vi "I2C and GPIO Timestamp Loop.vi"(0 "fpga interface in":refnum<k20>, 1 "'stop' notifier":refnum<notifier>, 2 "log to disk":bool=TRUE, 5 "tdms file directory":path, 7 "gpio to display":T2[](array[typedef])=[{"GPIO Bank"=enum."Ser0 GPIO Bank", "GPIO Number"=0}], 9 "timestamp filter":T1[](array[typedef])=[enum."User24", enum."User25", enum."User26", enum."User27", enum."User28", enum."User29", enum."User30", enum."User31"], 11 "error in (no error)":errorcluster) -> (4 "i2c data":string[][](array[string]), 6 "gpio timestamps waveform":digitalwaveform[](graph), 8 "error parsing gpio timestamps":bool, 15 "error out":errorcluster)   [LabVIEW 2023, in "GettingStarted_Common_148X_Host.lvlib"]
uses:
  GettingStarted_Common_148X_Host.lvlib
  <instrlib>/FlexRIO/CSI-2/v2/FPGA/Types/Timestamp ID.ctl
  <instrlib>/FlexRIO/CSI-2/v2/FPGA/NI CSI-2 API FPGA v2.lvlib
  Types/GPIO Filter.ctl
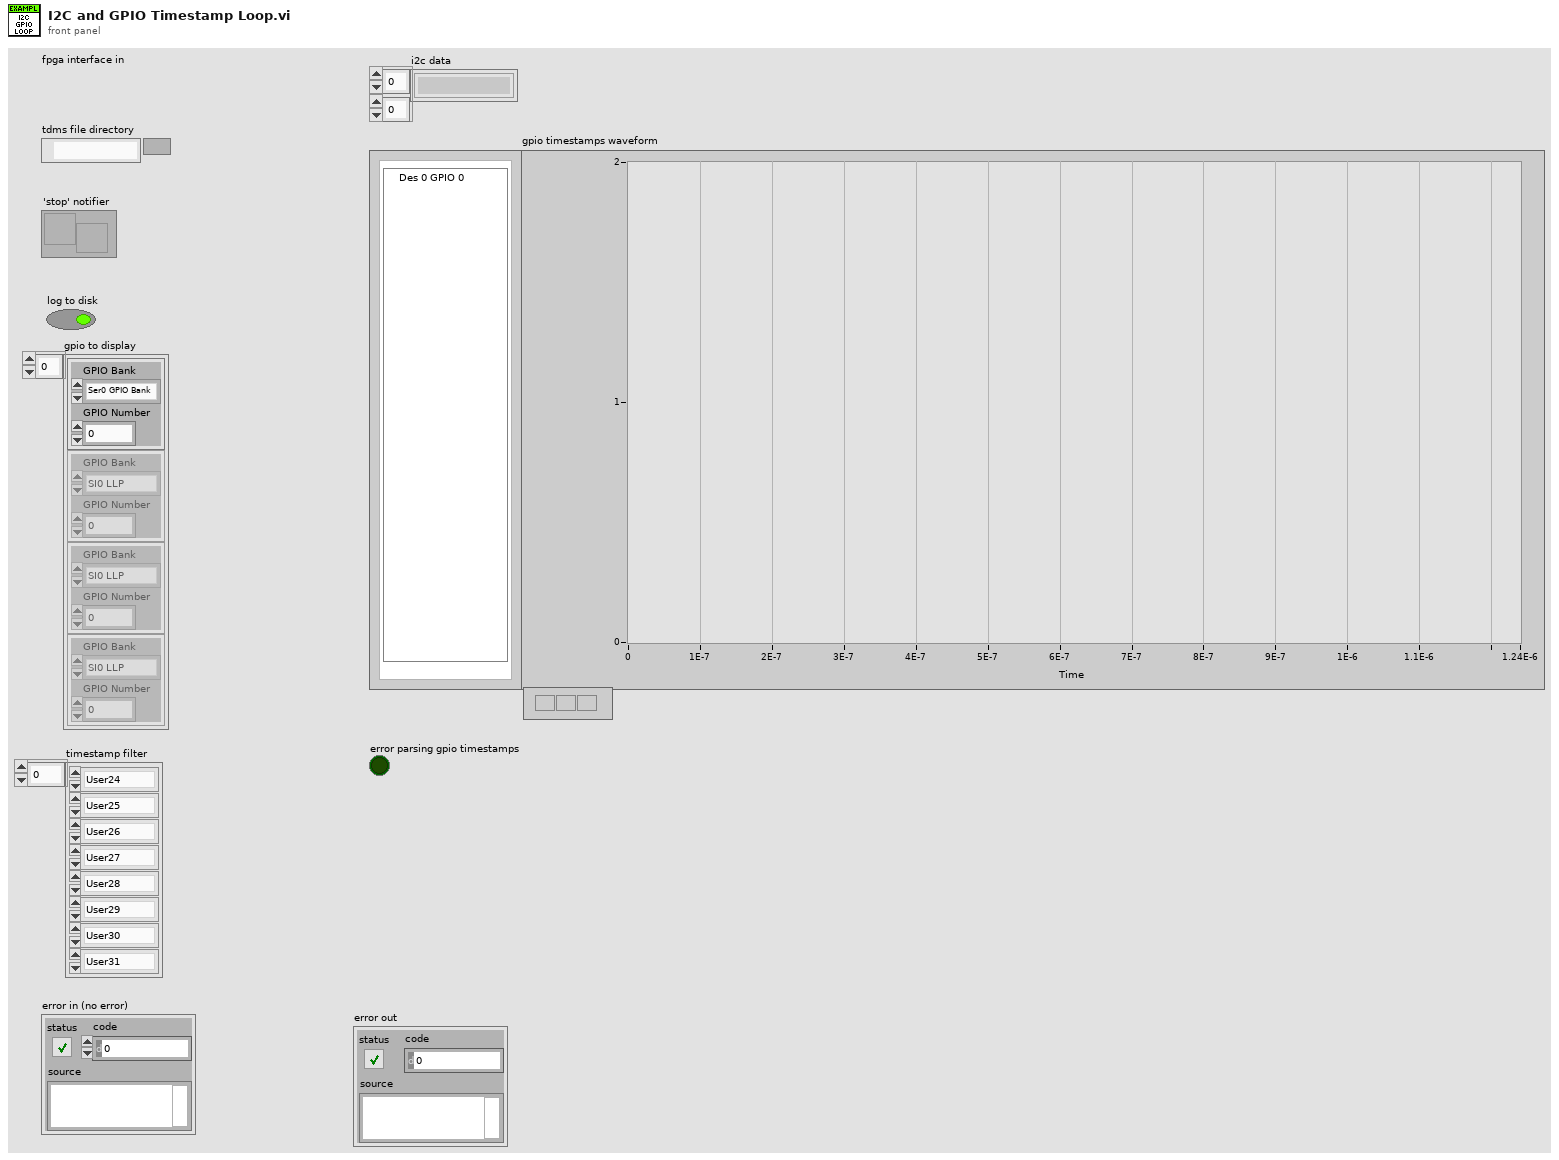
[diagram p1: front panel]
types:
  T1 = typedef "NI CSI-2 API FPGA v2.lvlib/Timestamp ID.ctl" = enum8{"SI0 LLP", "SI1 LLP", "SI2 LLP", "SI3 LLP", "SI4 LLP", "SI5 LLP", "SI6 LLP", "SI7 LLP", "SO0 LLP", "SO1 LLP", "SO2 LLP", "SO3 LLP", "SO4 LLP", "SO5 LLP", "SO6 LLP", "SO7 LLP", "Ser0 GPIO Bank", "Ser1 GPIO Bank", "Ser2 GPIO Bank", "Ser3 GPIO Bank", "Ser4 GPIO Bank", "Ser5 GPIO Bank", "Ser6 GPIO Bank", "Ser7 GPIO Bank", "Des0 GPIO Bank", "Des1 GPIO Bank", "Des2 GPIO Bank", "Des3 GPIO Bank", "Des4 GPIO Bank", "Des5 GPIO Bank", "Des6 GPIO Bank", "Des7 GPIO Bank", "User0", "User1", "User2", "User3", "User4", "User5", "User6", "User7", "User8", "User9", "User10", "User11", "User12", "User13", "User14", "User15", "User16", "User17", "User18", "User19", "User20", "User21", "User22", "User23", "User24", "User25", "User26", "User27", "User28", "User29", "User30", "User31"}
  T2 = typedef "GettingStarted_Common_148X_Host.lvlib/GPIO Filter.ctl" = cluster{"GPIO Bank":T1, "GPIO Number":i32}
  T3 = typedef "NI CSI-2 API FPGA v2.lvlib/User Timestamp.ctl" = cluster{"valid":bool, "user data":fxp<+,58,58>, "id":T1}
  T4 = typedef "NI CSI-2 API Host v2.lvlib/Host GPIO Bank Timestamp.ctl" = cluster{"valid":bool, "count":u64, "id":T1, "gpio bank":T5}
  T5 = typedef "NI CSI-2 API FPGA v2.lvlib/GPIO Bank.ctl" = cluster{"GPIO 0":bool, "GPIO 1":bool, "GPIO 2":bool, "GPIO 3":bool, "GPIO 4":bool, "GPIO 5":bool, "GPIO 6":bool, "GPIO 7":bool, "GPIO 8":bool, "GPIO 9":bool, "GPIO 10":bool}
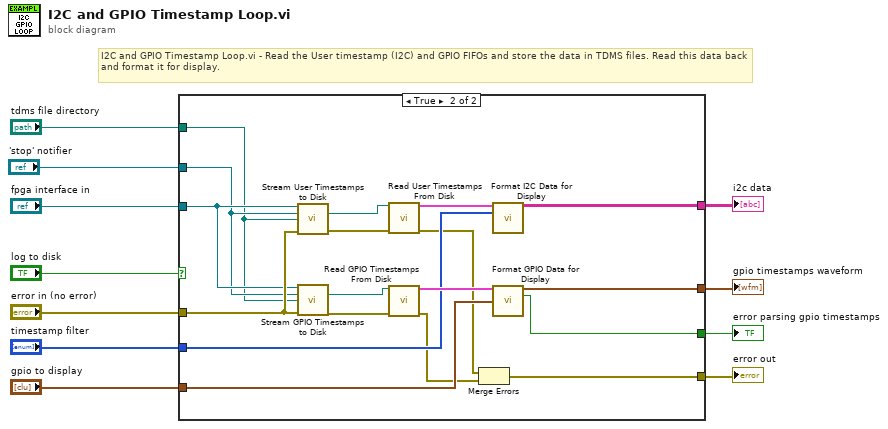
[diagram p0: block diagram]
diagram:
  # "I2C and GPIO Timestamp Loop.vi - Read the User timestamp (I2C) and GPIO FIFOs and store the data in TDMS files. Read this data back and format it for display."
  n1 = case shown="True" "log to disk" {
    tunnel: "error in (no error)" -> [w12 w30]
    tunnel: "fpga interface in" -> [_ w29]
    tunnel: "'stop' notifier" -> [_ w28]
    tunnel: "tdms file directory" -> [_ w27]
    tunnel: "gpio to display" -> [_ w26]
    tunnel: "timestamp filter" -> [_ w19]
    tunnel: [_ w16] -> w5
    tunnel: [_ w15] -> w4
    tunnel: [_ w14] -> w3
    tunnel: [w12 w13] -> w2
    frame False {
    }
    frame True {
      n2 = call "Stream User Timestamps to Disk.vi"("fpga interface in"=w29, "'stop' notifier"=w28, "base tdms file path"=w27, "error in (no error)"=w30) -> ("file path out"=w23:path, "error out"=w22:errorcluster)  [unwired: 8 in, 2 out]
      n3 = call "Stream GPIO Timestamps to Disk.vi"("fpga interface in"=w29, "'stop' notifier"=w28, "base tdms file path"=w27, "error in (no error)"=w30) -> ("file path out"=w25:path, "error out"=w24:errorcluster)  [unwired: 8 in, 2 out]
      n4 = call "Read User Timestamps From Disk.vi"("file path"=w23, "error in (no error)"=w22) -> ("user timestamps"=w20:T3[], "error out"=w18:errorcluster)  [unwired: 12 in]
      n5 = call "Read GPIO Timestamps From Disk.vi"("file path"=w25, "error in (no error)"=w24) -> ("gpio timestamps"=w21:T4[], "error out"=w17:errorcluster)  [unwired: 12 in]
      n6 = Merge Errors(w18, w17) -> (w13:errorcluster)
      n7 = call "Format I2C Data for Display.vi"("user timestamps"=w20, "timestamp filter"=w19) -> ("display data"=w14:string[][])  [unwired: 13 in]
      n8 = call "Format GPIO Data for Display.vi"("gpio timestamps"=w21, "gpio to display"=w26) -> ("gpio timestamps waveform"=w15:digitalwaveform[], "error parsing timestamps"=w16:bool)  [unwired: 12 in]
    }
  }
  "error out" <- w2
  "i2c data" <- w3
  "gpio timestamps waveform" <- w4
  "error parsing gpio timestamps" <- w5
